vi "LED Ctlr Cmds SA.vi"(0 "VISA session":refnum<visa-resource-name>="COM9", 5 "Intensity":dbl(knob) min=0.0 max=100.0 step=0.001 scale=0.0..100.0, 9 "Enable":u8=31, 11 "error in (no error)":errorcluster) -> (4 "VISA session out":refnum<visa-resource-name>, 6 "Bytes at port":u8, 8 "Response":string, 10 "Bytes Read":u8, 15 "error out":errorcluster)   [LabVIEW 2010]
uses:
  <vilib>/Instr/_visa.llb/VISA Configure Serial Port (Instr).vi
panel:
  in  "Stop":bool
  out "Intensity Set":u16
  in  "Serial Configuration":T1={"Baud Rate"=115200, "Parity"=0, "Data Bits"=8, "Stop Bits"=10, "Flow Control"=0} {"Flow Control" items=["None", "XON/XOFF", "RTS/CTS", "XON/XOFF & RTS/CTS", "DTR/DSR", "XON/XOFF & DTR/DSR"]; "Stop Bits" items=["1.0"=10, "1.5"=15, "2.0"=20]; "Data Bits" items=["7"=7, "8"=8]; "Parity" items=["None", "Odd", "Even", "Mark", "Space"]; "Baud Rate" items=["300"=300, "600"=600, "1200"=1200, "2400"=2400, "4800"=4800, "9600"=9600, "19200"=19200]}
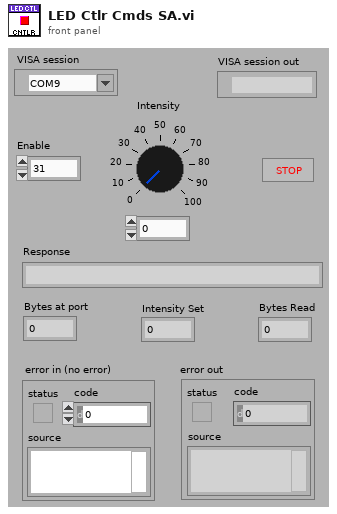
[diagram p1: front panel]
types:
  T1 = cluster{"Baud Rate":u32, "Parity":u16, "Data Bits":u16, "Stop Bits":u16, "Flow Control":u16}
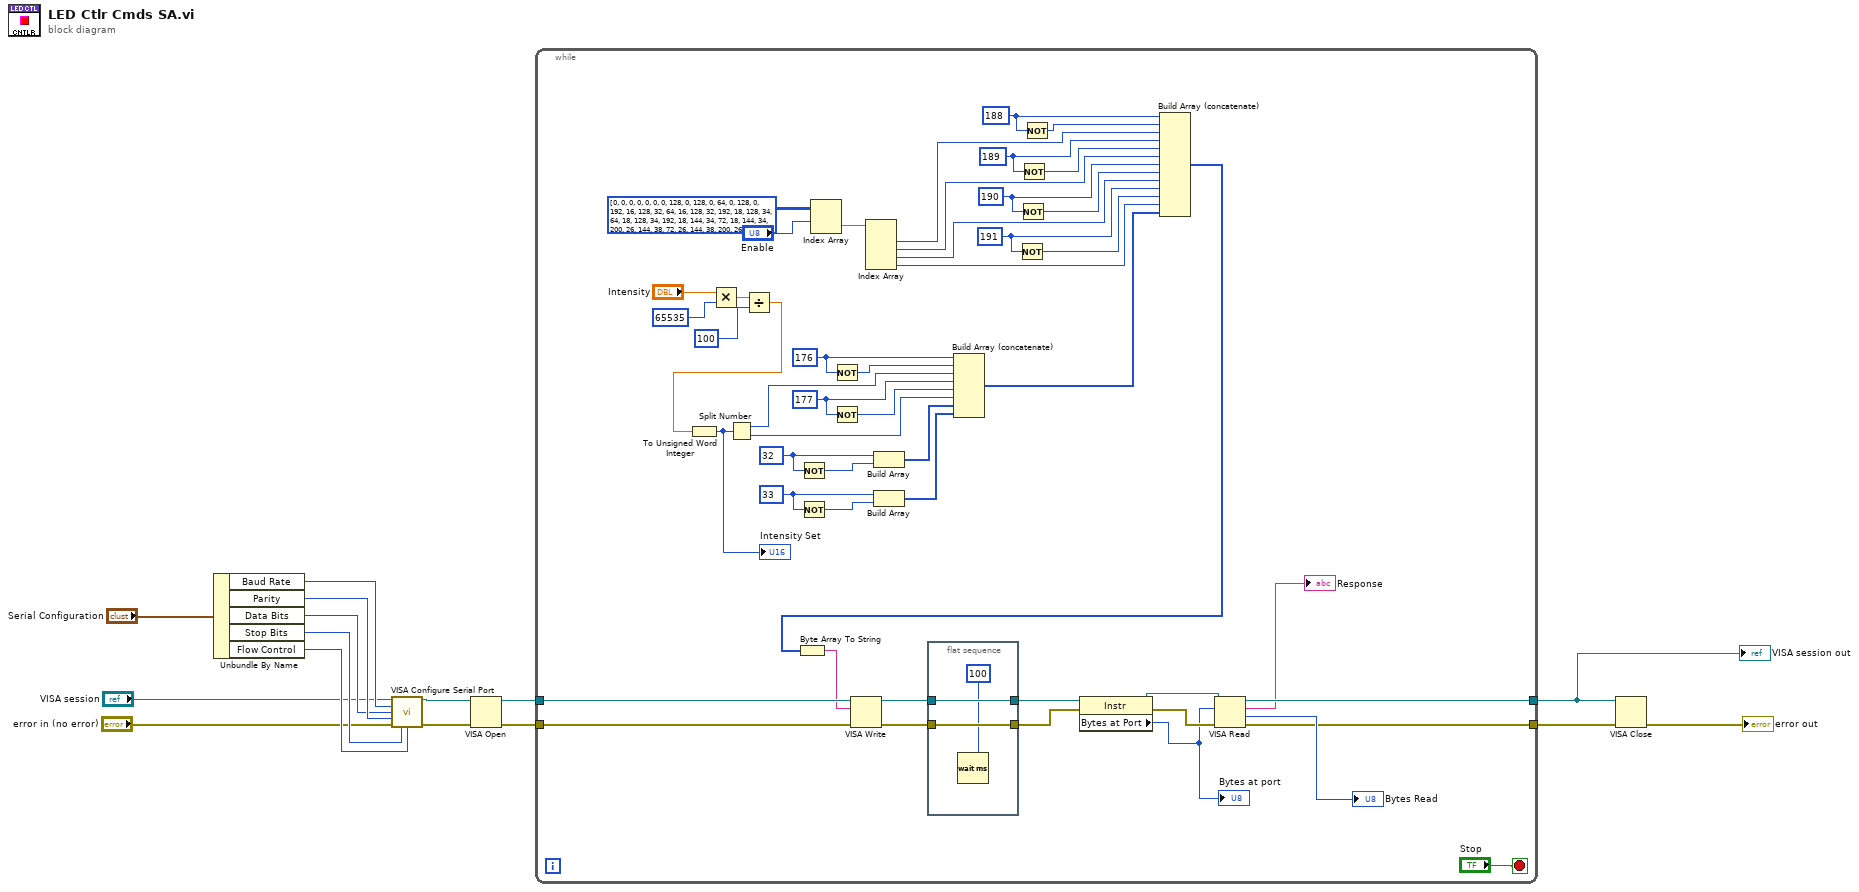
[diagram p0: block diagram]
diagram:
  n1 = Unbundle By Name("Serial Configuration") -> ("Baud Rate"=w14:u32, "Parity"=w13:u16, "Data Bits"=w12:u16, "Stop Bits"=w11:u16, "Flow Control"=w10:u16)
  n2 = call-poly "VISA Configure Serial Port"("VISA resource name"="VISA session", "baud rate (9600)"=w14, "data bits (8)"=w12, "parity (0:none)"=w13, "error in (no error)"="error in (no error)", "stop bits (10: 1 bit)"=w11, "flow control (0:none)"=w10) -> ("VISA resource name out"=w7:refnum<visa-resource-name>, "error out"=w6:errorcluster)  [unwired: 7 in]
  n3 = VISA Open(error in (no error)=w6, VISA resource name=w7) -> (VISA resource name=w5:refnum<visa-resource-name>, error out=w4:errorcluster)  [unwired: 3 in]
  n4 = while {
    tunnel: w5 -> [w65]
    tunnel: w4 -> [w64]
    tunnel: [w55] -> w3
    tunnel: [w54] -> w2
    stop <- "Stop" stop-if-true
    w26 = u8 33
    w30 = u8 32
    w34 = u8 177
    w37 = u8 176
    w41 = u8 191
    w43 = u8 190
    w46 = u8 189
    w50 = u8 188
    n5 = Multiply(x="Intensity", y=65535) -> (x*y=w20:dbl)
    n6 = Divide(x=w20, y=100) -> (x/y=w18:dbl)
    n7 = To Unsigned Word Integer(number=w18) -> (unsigned 16bit integer=w17:u16)
    "Intensity Set" <- w17
    n8 = Split Number(x=w17) -> (hi(x)=w35:u8, lo(x)=w32:u8)
    n9 = Not(x=w30) -> (.not. x?=w29:u8)
    n10 = Not(x=w26) -> (.not. x?=w27:u8)
    n11 = Index Array(array=u8[][] [[0, 0, 0, 0], [0, 0, 0, 128], [0, 128, 0, 64], [0, 128, 0, 192], [16, 128, 32, 64], [16, 128, 32, 192], [18, 128, 34, 64], [18, 128, 34, 192], [18, 144, 34, 72], [18, 144, 34, 200], [26, 144, 38, 72], [26, 144, 38, 200], [26, 208, 38, 88], [26, 208, 38, 216], [26, 216, 38, 92], [26, 216, 38, 220], [90, 216, 54, 92], [90, 216, 54, 220], [91, 216, 55, 92], [91, 216, 55, 220], [91, 218, 55, 93], [91, 218, 55, 221], [219, 218, 119, 93], [219, 218, 119, 221], [219, 222, 119, 95], [219, 222, 119, 223], [251, 222, 247, 95], [251, 222, 247, 223], [251, 254, 247, 127], [251, 254, 247, 255], [255, 254, 255, 127], [255, 255, 255, 255]], index (row)="Enable") -> (element=w48:u8[])  [unwired: 1 in]
    n12 = Not(x=w37) -> (.not. x?=w36:u8)
    n13 = Not(x=w34) -> (.not. x?=w33:u8)
    n14 = Index Array(array=w48) -> (element #1=w47:u8, element #2=w44:u8, element #3=w39:u8, element #4=w38:u8)  [unwired: 4 in]
    n15 = Build Array(w30, w29) -> (w28:u8[])
    n16 = Build Array(w26, w27) -> (w25:u8[])
    n17 = flat-sequence {
      tunnel: [w68] -> w61
      tunnel: w62 -> [w68]
      tunnel: [w67] -> w60
      tunnel: w63 -> [w67]
      frame #0 {
        n18 = Wait (ms)(milliseconds to wait=100) -> ()  [unwired: 1 out]
      }
    }
    n19 = Build Array (concatenate)(w37, w36, w35, w34, w33, w32, w28, w25) -> (w24:u8[])
    n20 = Not(x=w41) -> (.not. x?=w40:u8)
    n21 = Not(x=w43) -> (.not. x?=w42:u8)
    n22 = Not(x=w46) -> (.not. x?=w45:u8)
    n23 = Not(x=w50) -> (.not. x?=w49:u8)
    n24 = property class="Instr"(reference=w61, error in=w60) -> (reference out=w59:refnum<visa-resource-name>, error out=w58:errorcluster, "Bytes at Port"=w57:u32)
    "Bytes at port" <- w57
    n25 = Build Array (concatenate)(w50, w49, w47, w46, w45, w44, w43, w42, w39, w41, w40, w38, w24) -> (w23:u8[])
    n26 = Byte Array To String(unsigned byte array=w23) -> (string=w31:string)
    n27 = VISA Write(VISA resource name=w65, write buffer=w31, error in (no error)=w64) -> (VISA resource name out=w62:refnum<visa-resource-name>, error out=w63:errorcluster)  [unwired: 1 out]
    n28 = VISA Read(VISA resource name=w59, byte count=w57, error in (no error)=w58) -> (VISA resource name out=w54:refnum<visa-resource-name>, read buffer=→"Response":string, return count=→"Bytes Read":u32, error out=w55:errorcluster)
  }
  "VISA session out" <- w2
  n29 = VISA Close(VISA resource name=w2, error in (no error)=w3) -> (error out=→"error out":errorcluster)
